vi "Write Trigger Core.vi"(8 "error in (no error)":errorcluster, 10 "PV":refnum<class "PV.lvclass">, 11 "SVConnection in":refnum<class "SVConnection.lvclass">) -> (0 "error out":errorcluster, 3 "SVConnection out":refnum<class "SVConnection.lvclass">)   [LabVIEW 2015, in "CS++SharedVariables.lvlib" / "SVConnection.lvclass"]
doc: "Publish a process variable to trigger a paramater less message."
uses:
  SVConnection.lvclass
  ProcessVariable/PV.lvclass
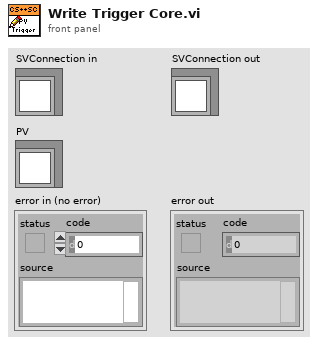
[diagram p1: front panel]
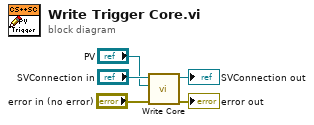
[diagram p0: block diagram]
diagram:
  n1 = call-dynamic "Write Core.vi"("error in (no error)"="error in (no error)", "PV"="PV", "PVConnection in"="SVConnection in") -> ("error out"=→"error out":errorcluster, "PVConnection out"=→"SVConnection out":refnum<class "SVConnection.lvclass">)  [unwired: 7 in]
